vi "Check_Device_Status.vi"(6 "Queues":T1, 7 "Main parameters in":T2={"Mode"={"Mode"=enum."Dialog", "Expert?"=FALSE, "Dialog?"=FALSE}, "Stop loop"={"Settings changed?"=FALSE, "Stop?"=refnum}, "Send message"={"Send mode"=enum."Get parameters", "Set parameter list"=0, "Get parameter list"=0, "Reset device"=0, "Length set settings message"=0, "Reset buttons?"=FALSE, "Reset Master?"=enum."General"}, "Write settings"={"Options"=enum."File 1"}, "Settings state"={"MAS locked?"=refnum, "SLV locked?"=refnum}, "Button refs"={"Stop program"=refnum, "Save settings"=refnum, "DAQ mode"=refnum, "Reset settings"=refnum, "Apply settings"=refnum, "Reset MAS"=refnum, "Reset SLV"=refnum, "Local DBase?"=refnum, "Last value DBase"=FALSE, "Database"=refnum, "Calibration"=refnum, "Save settings 2"=refnum}, "Update screen"={"Detector number"=0, "Hardware"=enum."None"}, "Files"={"Path config file"=path "", "Path def. ini file"=path "", "Path ini file 1"=path "", "Path ini file 2"=path "", "Path RBF file"=path ""}, "DB connection"={"connection reference"=refnum, "Connected?"=refnum, "ODBC Name"=""}, "Status_id"=refnum, "Time difference"=refnum, "Satellites"=refnum, "Alignment parameters"=refnum, "Page Statistics 2"=refnum, "Database"=refnum, "Page Statistics"=refnum} {"Update screen"."Detector number" format="%#.0f"; "Send message"."Reset device" format="%x"; "Send message"."Get parameter list" format="%x"; "Send message"."Set parameter list" format="%x"}, 8 "Status/Errors in":refnum<vi>, 9 "Control Parameters [] in":T16[](array[typedef]) {"Aux Byte Value" format="%02x"; "Max Real Value" format="%#_6e"; "Min Real Value" format="%#_6e"; "dReal/dByte" format="%#_6e"; "Byte Value" format="%02x"; "Identifier" format="%02x"}, 10 "Timer parameters in":refnum<vi>, 11 "Device in":refnum<vi>) -> (0 "Status/Errors out":refnum<vi>, 1 "Control Parameters [] out":T16[](array[typedef]) {"Aux Byte Value" format="%02x"; "Max Real Value" format="%#_6e"; "Min Real Value" format="%#_6e"; "dReal/dByte" format="%#_6e"; "Byte Value" format="%02x"; "Identifier" format="%02x"}, 2 "Timer parameters out":refnum<vi>, 3 "Device out":refnum<vi>, 5 "Main parameters out":T2={"Mode"={"Mode"=enum."Dialog", "Expert?"=FALSE, "Dialog?"=FALSE}, "Stop loop"={"Settings changed?"=FALSE, "Stop?"=refnum}, "Send message"={"Send mode"=enum."Get parameters", "Set parameter list"=0, "Get parameter list"=0, "Reset device"=0, "Length set settings message"=0, "Reset buttons?"=FALSE, "Reset Master?"=enum."General"}, "Write settings"={"Options"=enum."File 1"}, "Settings state"={"MAS locked?"=refnum, "SLV locked?"=refnum}, "Button refs"={"Stop program"=refnum, "Save settings"=refnum, "DAQ mode"=refnum, "Reset settings"=refnum, "Apply settings"=refnum, "Reset MAS"=refnum, "Reset SLV"=refnum, "Local DBase?"=refnum, "Last value DBase"=FALSE, "Database"=refnum, "Calibration"=refnum, "Save settings 2"=refnum}, "Update screen"={"Detector number"=0, "Hardware"=enum."None"}, "Files"={"Path config file"=path "", "Path def. ini file"=path "", "Path ini file 1"=path "", "Path ini file 2"=path "", "Path RBF file"=path ""}, "DB connection"={"connection reference"=refnum, "Connected?"=refnum, "ODBC Name"=""}, "Status_id"=refnum, "Time difference"=refnum, "Satellites"=refnum, "Alignment parameters"=refnum, "Page Statistics 2"=refnum, "Database"=refnum, "Page Statistics"=refnum} {"Update screen"."Detector number" format="%#.0f"; "Send message"."Reset device" format="%x"; "Send message"."Get parameter list" format="%x"; "Send message"."Set parameter list" format="%x"})   [LabVIEW 2010]
uses:
  Controls/Control_Parameters.ctl
  Controls/Master.ctl
  Controls/Main_Parameters.ctl
  Controls/Mode.ctl
  Controls/Stop_Loop.ctl
  Controls/Send_Message.ctl
  Controls/Send_Message_Mode.ctl
  Controls/Write_Settings.ctl
  Controls/Write_Settings_Options.ctl
  Controls/Settings_State.ctl
  Controls/Button_Refs.ctl
  Controls/Update_Screen.ctl
  Controls/Files.ctl
  Controls/DB_Connection.ctl
  database/Connection.llb/Conn ObjectReference.ctl
  Controls/Queues.ctl
  Controls/One_Second.ctl
  Controls/GPS_Timestamp.ctl
  Controls/Device_Elements.ctl
  Controls/Get_Set_Device_Options.ctl
  Controls/Get_Set_Settings_State_Options.ctl
  Controls/Get_Set_Timer_Options.ctl
  Controls/Get_Set_Connection_Options.ctl
  Controls/Get_Set_Buttons_mode.ctl
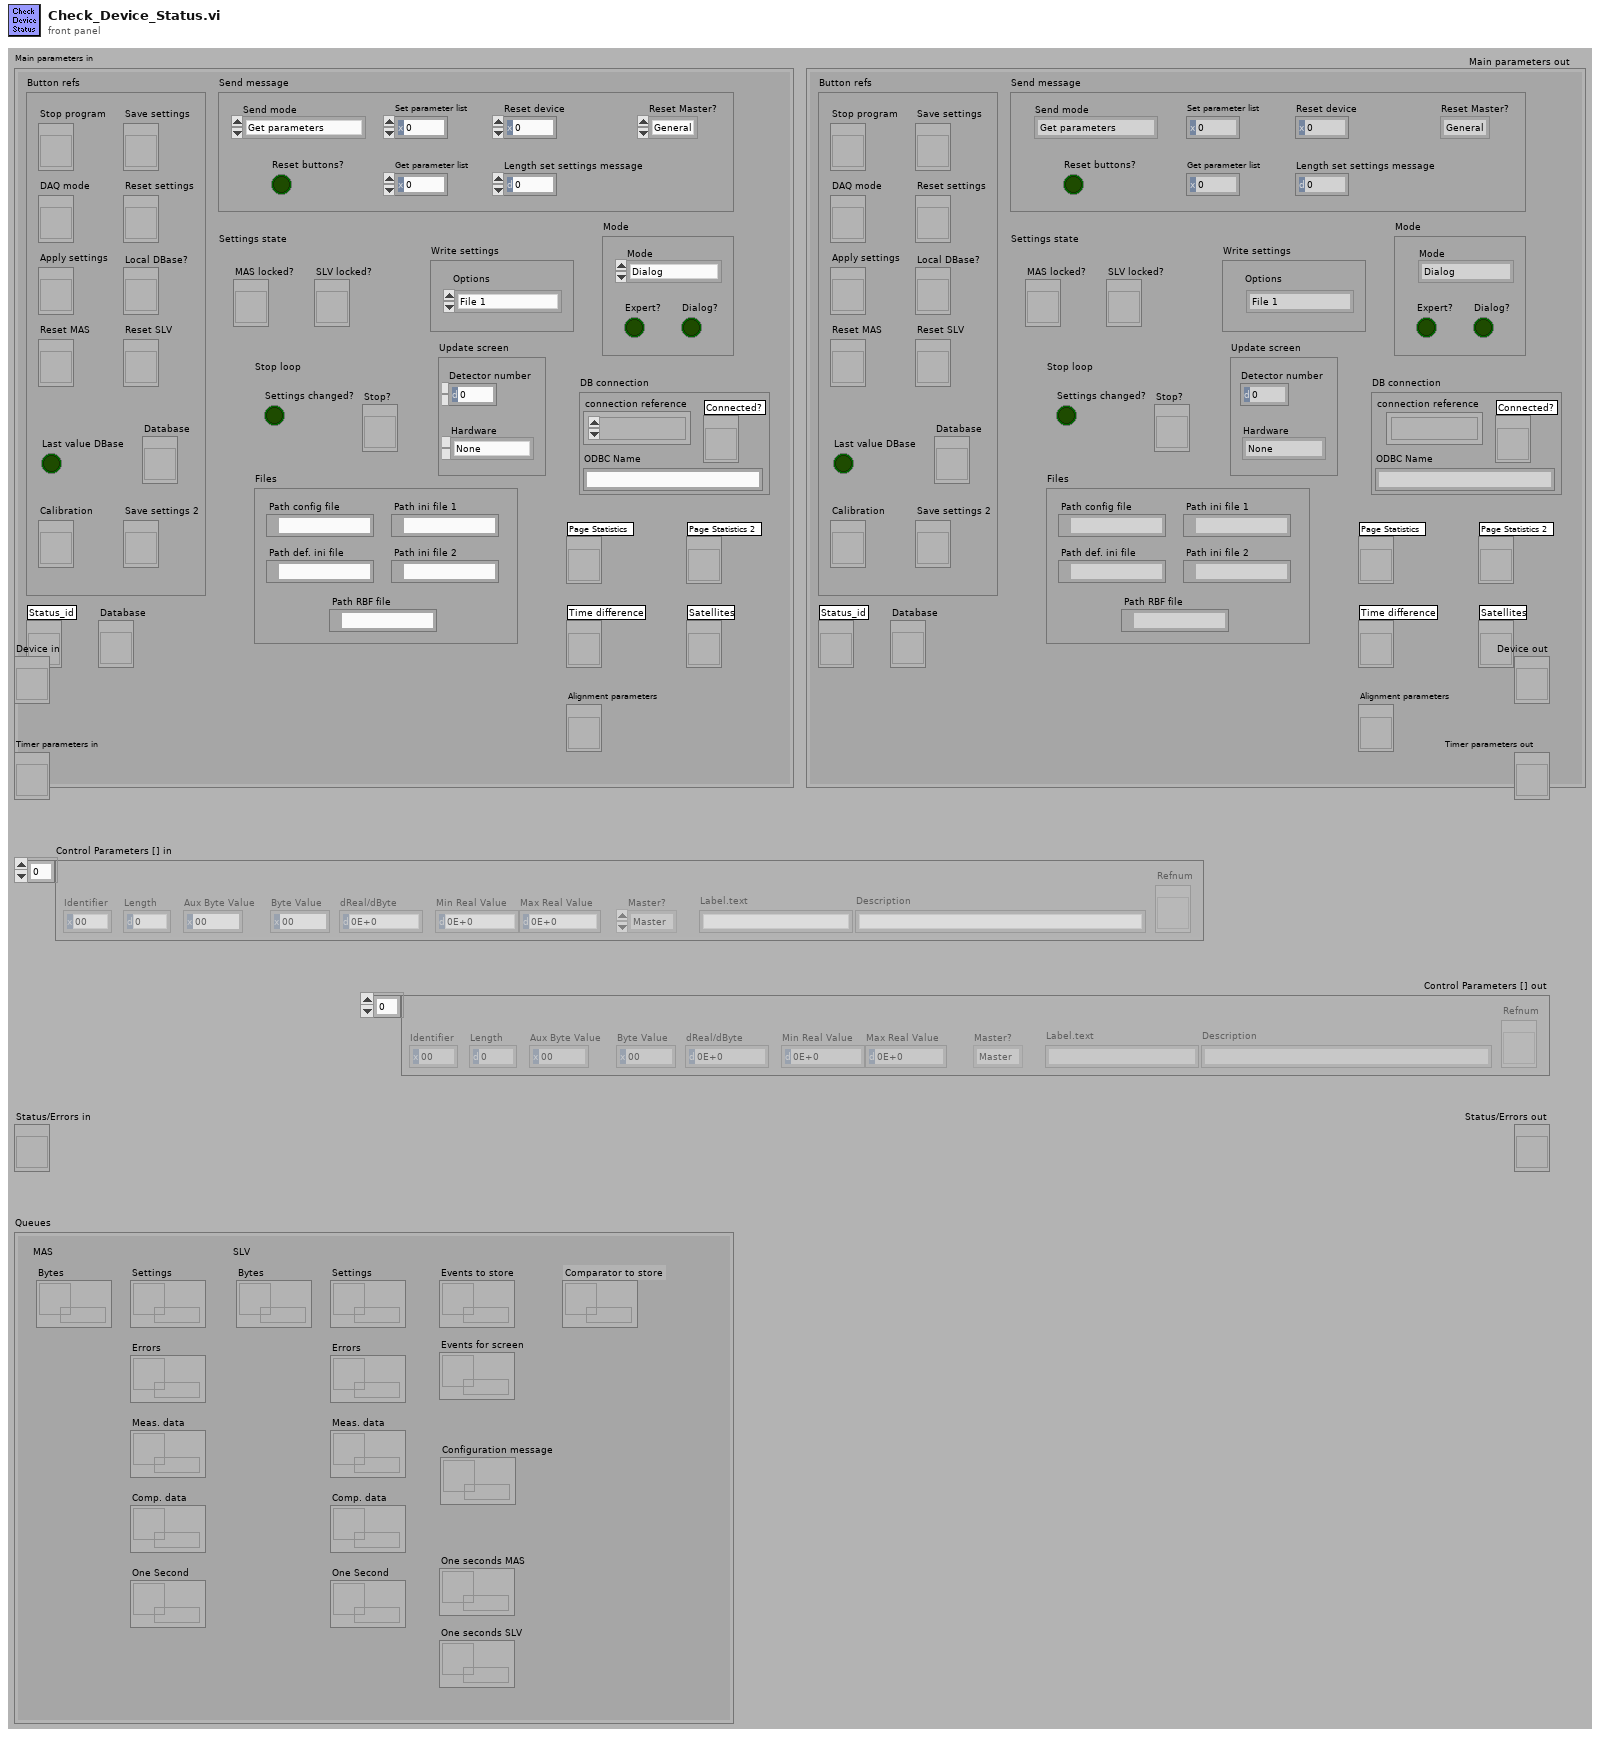
[diagram p1: front panel]
types:
  T1 = typedef "Queues.ctl" = cluster{"MAS":cluster{"Bytes":refnum<queue>, "Settings":refnum<queue>, "Errors":refnum<queue>, "Meas. data":refnum<queue>, "One Second":refnum<queue>, "Comp. data":refnum<queue>}, "SLV":cluster{"Bytes":refnum<queue>, "Settings":refnum<queue>, "Errors":refnum<queue>, "Meas. data":refnum<queue>, "One Second":refnum<queue>, "Comp. data":refnum<queue>}, "Events to store":refnum<queue>, "Events for screen":refnum<queue>, "One seconds MAS":refnum<queue>, "One seconds SLV":refnum<queue>, "Configuration message":refnum<queue>, "Comparator to store":refnum<queue>}
  T2 = typedef "Main_Parameters.ctl" = cluster{"Mode":T3, "Stop loop":T4, "Send message":T5, "Write settings":T8, "Settings state":T10, "Button refs":T11, "Update screen":T12, "Files":T13, "DB connection":T14, "Status_id":refnum<vi>, "Time difference":refnum<vi>, "Satellites":refnum<vi>, "Alignment parameters":refnum<vi>, "Page Statistics 2":refnum<vi>, "Database":refnum<vi>, "Page Statistics":refnum<vi>}
  T3 = typedef "Mode.ctl" = cluster{"Mode":enum8{"Stop", "Dialog", "Hisparc II", "Hisparc II DAQ", "Alignment"}, "Expert?":bool, "Dialog?":bool}
  T4 = typedef "Stop_Loop.ctl" = cluster{"Settings changed?":bool, "Stop?":refnum<vi>}
  T5 = typedef "Send_Message.ctl" = cluster{"Send mode":T6, "Set parameter list":u8, "Get parameter list":u8, "Reset device":u8, "Length set settings message":i32, "Reset buttons?":bool, "Reset Master?":T7}
  T6 = typedef "Send_Message_Mode.ctl" = enum16{"Get parameters", "Set parameters", "From front panel", "From parameters", "Reset device", "Alignment"}
  T7 = typedef "Master.ctl" = enum16{"Master", "Slave", "General"}
  T8 = typedef "Write_Settings.ctl" = cluster{"Options":T9}
  T9 = typedef "Write_Settings_Options.ctl" = enum16{"File 1", "File 2", "Alignment", "Reset"}
  T10 = typedef "Settings_State.ctl" = cluster{"MAS locked?":refnum<vi>, "SLV locked?":refnum<vi>}
  T11 = typedef "Button_Refs.ctl" = cluster{"Stop program":refnum<vi>, "Save settings":refnum<vi>, "DAQ mode":refnum<vi>, "Reset settings":refnum<vi>, "Apply settings":refnum<vi>, "Reset MAS":refnum<vi>, "Reset SLV":refnum<vi>, "Local DBase?":refnum<vi>, "Last value DBase":bool, "Database":refnum<vi>, "Calibration":refnum<vi>, "Save settings 2":refnum<vi>}
  T12 = typedef "Update_Screen.ctl" = cluster{"Detector number":u16, "Hardware":enum8{"None", "HiSPARC I", "HiSPARC II", "HiSPARC III", "Unknown"}}
  T13 = typedef "Files.ctl" = cluster{"Path config file":path, "Path def. ini file":path, "Path ini file 1":path, "Path ini file 2":path, "Path RBF file":path}
  T14 = typedef "DB_Connection.ctl" = cluster{"connection reference":T15, "Connected?":refnum<vi>, "ODBC Name":string}
  T15 = typedef "Conn ObjectReference.ctl" = refnum<k1>
  T16 = typedef "Control_Parameters.ctl" = cluster{"Identifier":u8, "Length":u16, "Byte Value":u32, "dReal/dByte":dbl, "Min Real Value":dbl, "Max Real Value":dbl, "Master?":T7, "Label.text":string, "Description":string, "Refnum":refnum<vi>, "Aux Byte Value":u32}
  T17 = typedef "Get_Set_Settings_State_Options.ctl" = enum16{"Get", "Lock", "Unlock"}
  T18 = typedef "Get_Set_Device_Options.ctl" = enum16{"Get", "Get cluster", "Set"}
  T19 = typedef "Device_Elements.ctl" = enum16{"Default", "Master?", "Connected?", "Status", "Disconnect?", "Handle", "Version number"}
  T20 = typedef "Device.ctl" = cluster{"Master?":T7, "Connected?":bool, "Status":bool, "Disconnect?":bool, "Handle":u32, "Version number":u32}
  T21 = typedef "Get_Set_Timer_Options.ctl" = enum16{"Get", "Get cluster", "Set", "Set to current time"}
  T22 = typedef "Timer_Parameters.ctl" = cluster{"current time (ms)":u32, "time (ms) screen updated":u32, "time (ms) controls locked":u32, "time (ms) last device check":u32, "time (ms) last data MAS":u32, "time (ms) last data SLV":u32, "time (ms) bad status MAS":u32, "time (ms) bad status SLV":u32, "time (ms) clock error updated":u32, "time delay screen update (ms)":u32, "time delay controls (ms)":u32, "time delay device check (ms)":u32, "time until MAS status bad (ms)":u32, "time until SLV status bad (ms)":u32, "time until MAS connection bad (ms)":u32, "time until SLV connection bad (ms)":u32, "time delay clock error update (ms)":u32}
  T23 = typedef "Get_Set_Connection_Options.ctl" = enum16{"Get", "Set connect", "Set disconnect"}
  T24 = typedef "Get_Set_Buttons_mode.ctl" = enum16{"Get", "Get DAQ", "Set", "Set settings"}
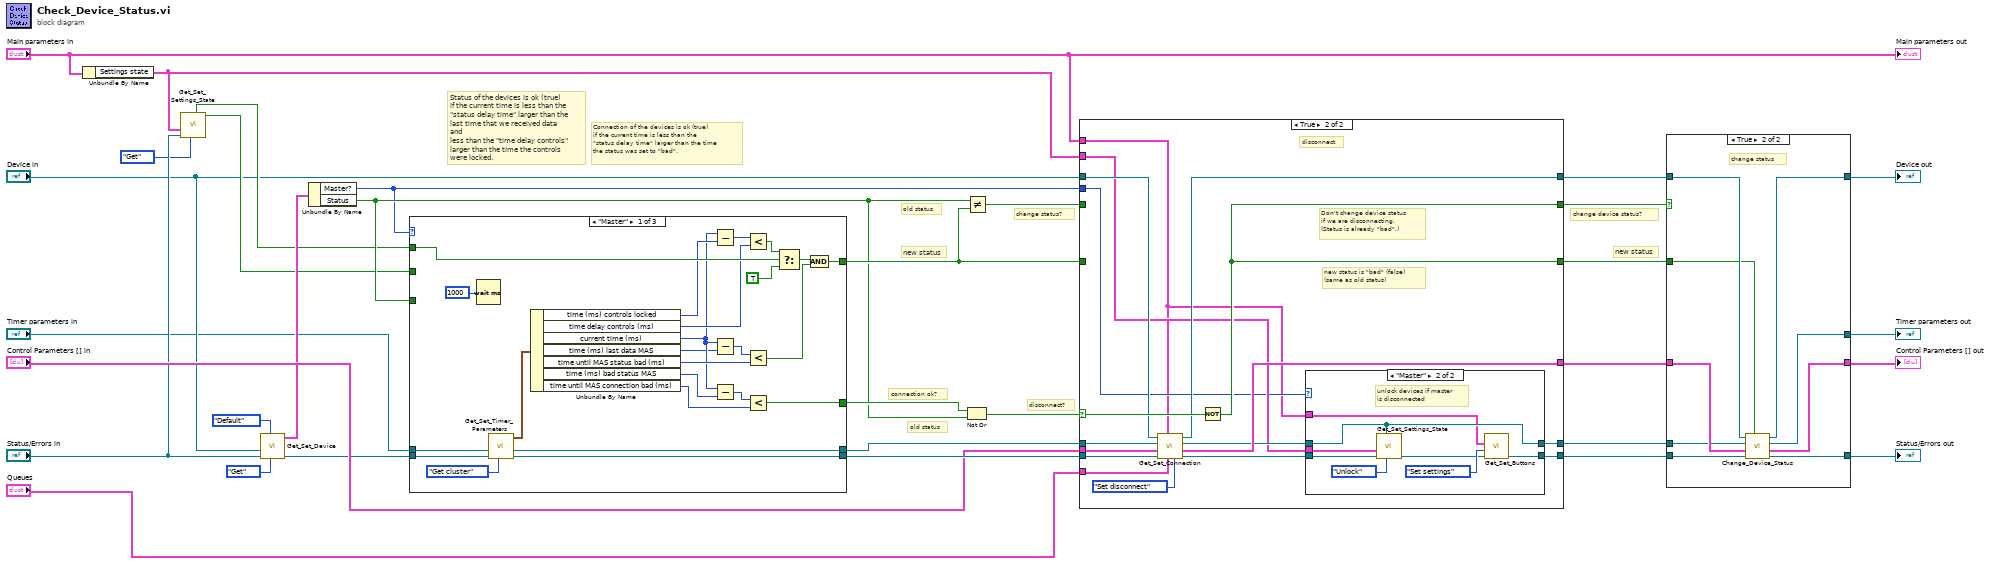
[diagram p0: block diagram]
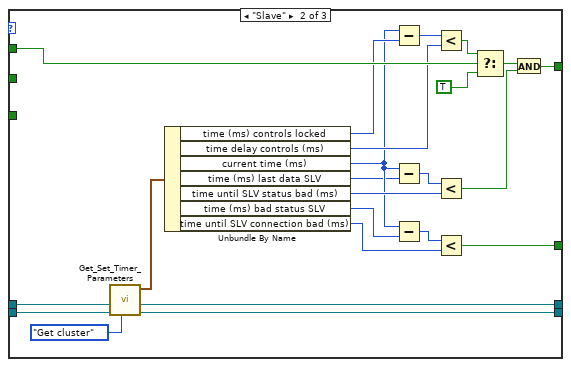
[diagram p4: hidden frame]
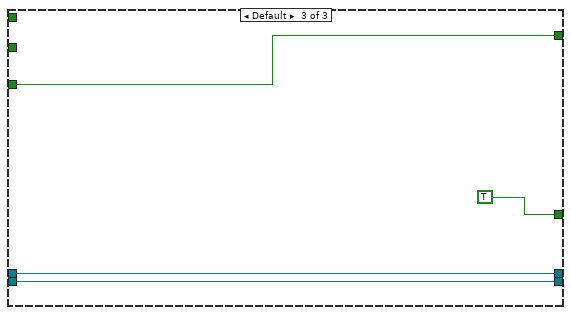
[diagram p5: hidden frame]
diagram:
  # "Connection of the devices is ok (true)\nif the current time is less than the\n\"status delay time\" larger than the time\nthe status was set to \"bad\"."
  # "old status"
  # "old status"
  # "new status"
  # "change device status?"
  # "disconnect?"
  # "change status?"
  # "connection ok?"
  # "new status"
  # "Status of the devices is ok (true)\nif the current time is less than the\n\"status delay time\" larger than the\nlast time that we received data and\nless than the \"time delay controls\"\nlarger than the time the controls\nwere locked."
  n1 = Unbundle By Name("Main parameters in") -> ("Settings state"=w6:T10)
  n2 = call "Get_Set_Settings_State.vi"("Get/Set"=Get_Set_Settings_State_Options."Get", "Status/Errors in"="Status/Errors in", "Settings state"=w6) -> ("SLV locked?"=w8:bool, "MAS locked?"=w9:bool)  [unwired: 2 in, 5 out]
  n3 = call "Get_Set_Device.vi"("Get/Set"=Get_Set_Device_Options."Get", "Element"=Device_Elements."Default", "Status/Errors in"="Status/Errors in", "Device in"="Device in") -> ("Status/Errors out"=w17:refnum<vi>, "Device"=w16:T20)  [unwired: 1 in, 5 out]
  n4 = Unbundle By Name(w16) -> ("Master?"=w7:T7, "Status"=w15:bool)
  n5 = case shown="\"Master\"" w7 {
    tunnel: "Timer parameters in" -> [w55 w78 w81]
    tunnel: [w51 w74 w83] -> w26
    tunnel: [w56 w79 TRUE] -> w30
    tunnel: w15 -> [_ _ w83]
    tunnel: w17 -> [w54 w77 w82]
    tunnel: [w53 w76 w82] -> w21
    tunnel: [w52 w75 w81] -> w18
    tunnel: w9 -> [w47 w70 _]
    tunnel: w8 -> [_ _ _]
    frame "Master" {
      n6 = Wait (ms)(milliseconds to wait=u32 1000) -> ()  [unwired: 1 out]
      n7 = call "Get_Set_Timer_Parameters.vi"("Get/Set"=Get_Set_Timer_Options."Get cluster", "Status/Errors in"=w54, "Timer parameters in"=w55) -> ("Status/Errors out"=w53:refnum<vi>, "Timer parameters out"=w52:refnum<vi>, "Timer cluster"=w46:T22)  [unwired: 2 in, 4 out]
      n8 = Unbundle By Name(w46) -> ("time (ms) controls locked"=w44:u32, "time delay controls (ms)"=w42:u32, "current time (ms)"=w35:u32, "time (ms) last data MAS"=w34:u32, "time until MAS status bad (ms)"=w41:u32, "time (ms) bad status MAS"=w39:u32, "time until MAS connection bad (ms)"=w38:u32)
      n9 = Subtract(x=w35, y=w44) -> (x-y=w43:u32)
      n10 = Subtract(x=w35, y=w34) -> (x-y=w36:u32)
      n11 = Subtract(x=w35, y=w39) -> (x-y=w40:u32)
      n12 = Less?(x=w43, y=w42) -> (x < y?=w48:bool)
      n13 = Less?(x=w36, y=w41) -> (x < y?=w37:bool)
      n14 = Less?(x=w40, y=w38) -> (x < y?=w56:bool)
      n15 = Select(t=w48, s=w47, f=TRUE) -> (s? t:f=w50:bool)
      n16 = And(x=w50, y=w37) -> (x .and. y?=w51:bool)
    }
    frame "Slave" {
      n17 = call "Get_Set_Timer_Parameters.vi"("Get/Set"=Get_Set_Timer_Options."Get cluster", "Status/Errors in"=w77, "Timer parameters in"=w78) -> ("Status/Errors out"=w76:refnum<vi>, "Timer parameters out"=w75:refnum<vi>, "Timer cluster"=w69:T22)  [unwired: 2 in, 4 out]
      n18 = Unbundle By Name(w69) -> ("time (ms) controls locked"=w67:u32, "time delay controls (ms)"=w65:u32, "current time (ms)"=w58:u32, "time (ms) last data SLV"=w57:u32, "time until SLV status bad (ms)"=w64:u32, "time (ms) bad status SLV"=w62:u32, "time until SLV connection bad (ms)"=w61:u32)
      n19 = Subtract(x=w58, y=w67) -> (x-y=w66:u32)
      n20 = Subtract(x=w58, y=w57) -> (x-y=w60:u32)
      n21 = Subtract(x=w58, y=w62) -> (x-y=w63:u32)
      n22 = Less?(x=w66, y=w65) -> (x < y?=w71:bool)
      n23 = Less?(x=w60, y=w64) -> (x < y?=w59:bool)
      n24 = Less?(x=w63, y=w61) -> (x < y?=w79:bool)
      n25 = Select(t=w71, s=w70, f=TRUE) -> (s? t:f=w73:bool)
      n26 = And(x=w73, y=w59) -> (x .and. y?=w74:bool)
    }
    frame Default {
    }
  }
  n27 = Not Or(1:w15, 2:w30) -> (0:w32:bool)
  n28 = Not Equal?(x=w15, y=w26) -> (x != y?=w27:bool)
  n29 = case shown="True" w32 {
    selector: w32 -> [_ w106]
    tunnel: "Device in" -> [w89 w103]
    tunnel: [w89 w102] -> w31
    tunnel: [w88 w105] -> w29
    tunnel: [w87 w105] -> w28
    tunnel: w27 -> [w88 _]
    tunnel: w26 -> [w87 _]
    tunnel: w21 -> [w86 w104]
    tunnel: [w86 w96] -> w23
    tunnel: "Control Parameters [] in" -> [w85 w101]
    tunnel: [w85 w100] -> w25
    tunnel: [w84 w92] -> w19
    tunnel: w18 -> [w84 w99]
    tunnel: "Queues" -> [_ w97]
    tunnel: w7 -> [_ w91]
    tunnel: w6 -> [_ w93]
    tunnel: "Main parameters in" -> [_ w90]
    frame False {
      # "do not disconnect"
    }
    frame True {
      # "disconnect"
      # "new status is \"bad\" (false)\n(same as old status)"
      # "Don't change device status\nif we are disconnecting.\n(Status is already \"bad\".)"
      n30 = call "Get_Set_Connection.vi"("Get/Set"=Get_Set_Connection_Options."Set disconnect", "Queues"=w97, "Main parameters in"=w90, "Status/Errors in"=w104, "Control Parameters [] in"=w101, "Timer parameters in"=w99, "Device in"=w103) -> ("Status/Errors out"=w95:refnum<vi>, "Control Parameters [] out"=w100:T16[], "Timer parameters out"=w94:refnum<vi>, "Device out"=w102:refnum<vi>)  [unwired: 1 out]
      n31 = Not(x=w106) -> (.not. x?=w105:bool)
      n32 = case shown="\"Master\"" w91 {
        tunnel: [w107 w111] -> w96
        tunnel: w95 -> [w107 w116]
        tunnel: w94 -> [w108 w110]
        tunnel: w93 -> [_ w114]
        tunnel: [w108 w110] -> w92
        tunnel: w90 -> [_ w109]
        frame Default {
        }
        frame "Master" {
          # "unlock devices if master\nis disconnected"
          n33 = call "Get_Set_Settings_State.vi"("Get/Set"=Get_Set_Settings_State_Options."Unlock", "Timer parameters"=w110, "Status/Errors in"=w116, "Settings state"=w114) -> ("Status/Errors out"=w112:refnum<vi>)  [unwired: 1 in, 6 out]
          n34 = call "Get_Set_Buttons.vi"("Status/Errors in"=w112, "Set?"=Get_Set_Buttons_mode."Set settings", "Main parameters"=w109) -> ("Status/Errors out"=w111:refnum<vi>)  [unwired: 8 out]
        }
      }
    }
  }
  n35 = case shown="True" w29 {
    tunnel: w25 -> [w118 w129]
    tunnel: w23 -> [w117 w125]
    tunnel: w28 -> [_ w123]
    tunnel: w31 -> [w120 w128]
    tunnel: [w120 w127] -> w3
    tunnel: w19 -> [w119 w122]
    tunnel: [w119 w121] -> w1
    tunnel: [w118 w126] -> w24
    tunnel: [w117 w124] -> w22
    frame False {
      # "do not change status"
    }
    frame True {
      # "change status"
      n36 = call "Change_Device_Status.vi"("New Status in"=w123, "Status/Errors in"=w125, "Control Parameters [] in"=w129, "Timer parameters in"=w122, "Device in"=w128) -> ("Status/Errors out"=w124:refnum<vi>, "Control Parameters [] out"=w126:T16[], "Timer parameters out"=w121:refnum<vi>, "Device out"=w127:refnum<vi>)  [unwired: 3 out]
    }
  }
  "Status/Errors out" <- w22
  "Control Parameters [] out" <- w24
  "Device out" <- w3
  "Timer parameters out" <- w1
  "Main parameters out" <- "Main parameters in"
